vi "电信1801-2018012704-杜兴安-虚拟仪器作业5.vi"() -> ()   [LabVIEW 2020]
uses:
  <vilib>/Analysis/2dsp.llb/Real FFT.vi
  <vilib>/measure/matone.llb/Harmonic Distortion Analyzer 1 Chan.vi
  <vilib>/measure/mascope.llb/Cycle Average and RMS 1 chan.vi
  <vilib>/measure/NI_MABase.lvlib
  <vilib>/measure/NI_MAPro.lvlib
  <vilib>/Analysis/NI_AALPro.lvlib
  <vilib>/Analysis/NI_AALBase.lvlib
panel:
  out "谐波幅值":dbl[](array[numeric])
  out "检测的基频值":dbl
  out "THD%":dbl
  in  "谐波次数":dbl=4.0
  in  "采样点数 6":dbl=1000.0
  in  "采样频率 6":dbl=1000.0
  in  "基频":dbl=50.0
  out "频谱":T1(graph)
  out "信号波形 2":waveform(dbl)(graph)
  in  "采样点数 5":dbl=100.0
  in  "采样频率 5":dbl=100.0
  in  "信号频率 3":dbl=5.0
  out "相位谱波形":T2(graph)
  out "幅度谱波形":T3(graph)
  out "信号波形":waveform(dbl)(graph)
  out "实际单频信号频率":dbl[](array[numeric])
  in  "采样信息":cluster{"采样频率":dbl, "采样点数":dbl}={"采样频率"=1000.0, "采样点数"=1000.0}
  in  "初始相位 2":dbl[](array[numeric])
  in  "幅值 2":dbl[](array[numeric]) format="%02_2g"
  in  "频率 2":dbl[](array[numeric])
  out "波形图 4":waveform(dbl)(graph)
  in  "采样点数 4":dbl=100.0
  in  "采样频率 4":dbl=100.0
  in  "幅值2":dbl=2.0
  in  "频率2":dbl=20.0
  in  "幅值1":dbl=1.0
  in  "频率1":dbl=10.0
  out "频域波形":cluster{i32, dbl, dbl[]}(graph)
  out "时域波形":cluster{i32, dbl, dbl[]}(graph)
  out "波形图 3":waveform(dbl)(graph)
  in  "采样点数 3":dbl=1000.0
  in  "采样频率 3":dbl=1000.0
  in  "公式":string="sin(w*t)/(w*t)"
  in  "幅值":dbl=1.0
  in  "频率":dbl=5.0
  out "波形图 2":waveform(dbl)(graph)
  in  "信号频率 2":dbl=5.0
  in  "信号幅度":dbl=1.0
  in  "初始相位":dbl
  in  "方波占空比":dbl=50.0
  in  "采样频率 2":dbl=1000.0
  in  "采样点数 2":dbl=1000.0
  in  "信号类型":u16(ring) items=["正弦波", "三角波", "方波", "锯齿波"]
  in  "停止 2":bool
  in  "信号幅值":dbl=1.0
  in  "信号频率":dbl=5.0
  in  "采样频率":dbl=1000.0
  in  "采样点数":dbl=1000.0
  out "波形图":waveform(dbl)(graph)
  in  "停止":bool
  out "周期平均值":sgl format="%04_1f"
  out "周期均方根":sgl format="%04_3g"
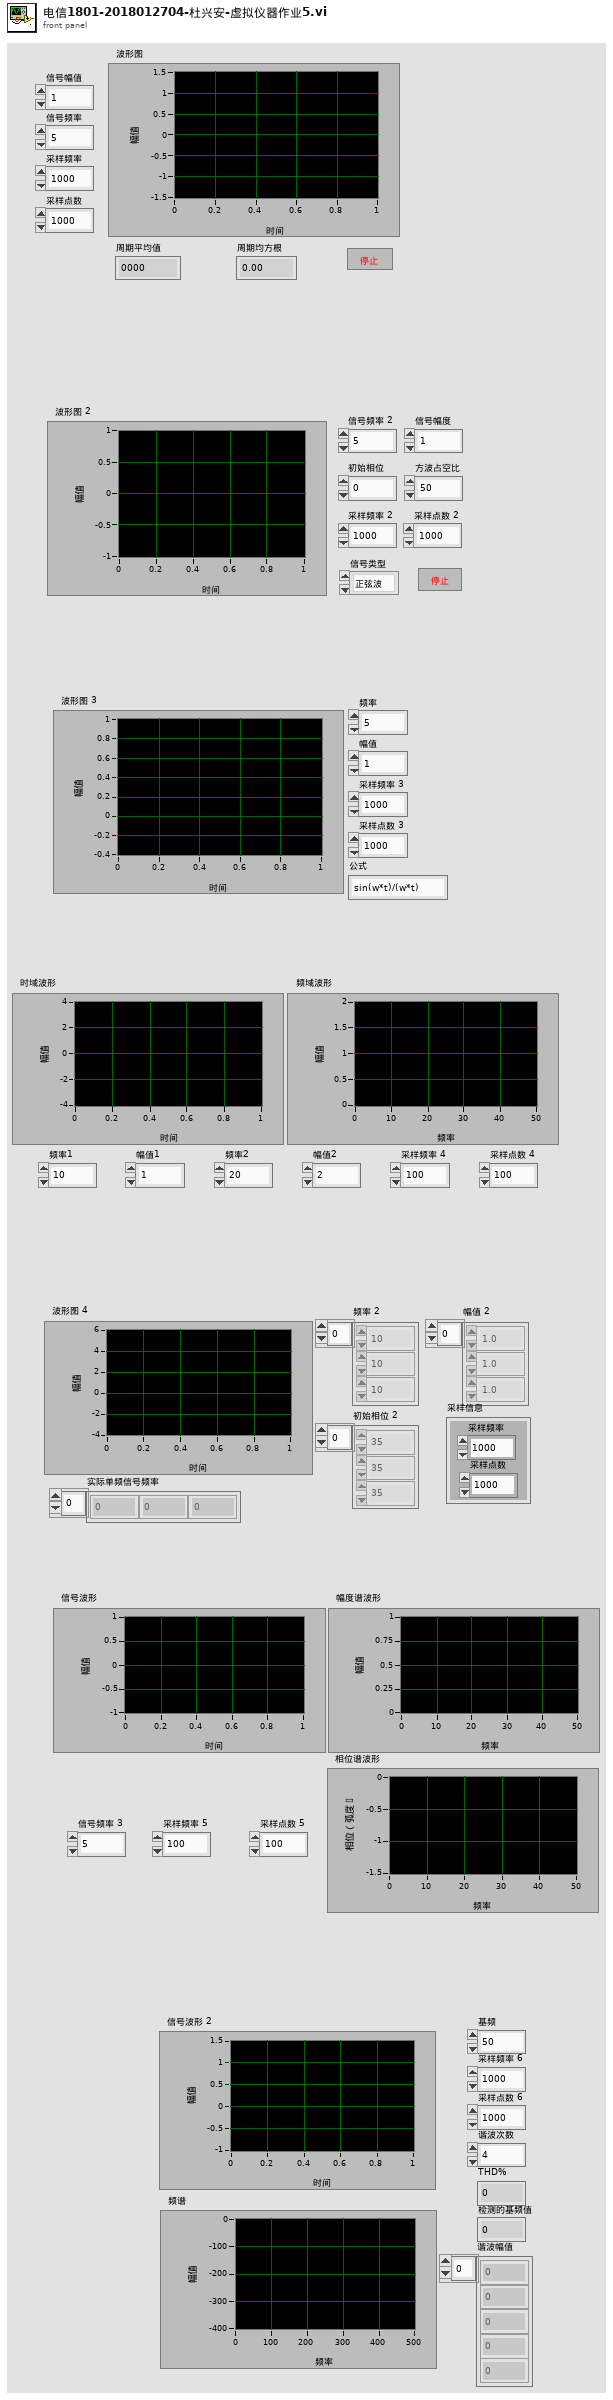
[diagram p1: front panel]
types:
  T1 = cluster{"f0":dbl, "df":dbl, "dB Spectrum (Hann)":dbl[]}
  T2 = cluster{i32, "df":dbl, "Amp Spectrum Phase (radians)":dbl[]}
  T3 = cluster{i32, "df":dbl, "Amp Spectrum Mag (Vrms)":dbl[]}
  T4 = enum16{"none", "input signal", "fundamental signal", "residual signal", "harmonics only", "noise and spurs"}
  T5 = cluster{"exported time signal":waveform(dbl), "exported spectrum (dB)":cluster{"f0":dbl, "df":dbl, "dB Spectrum (Hann)":dbl[]}}
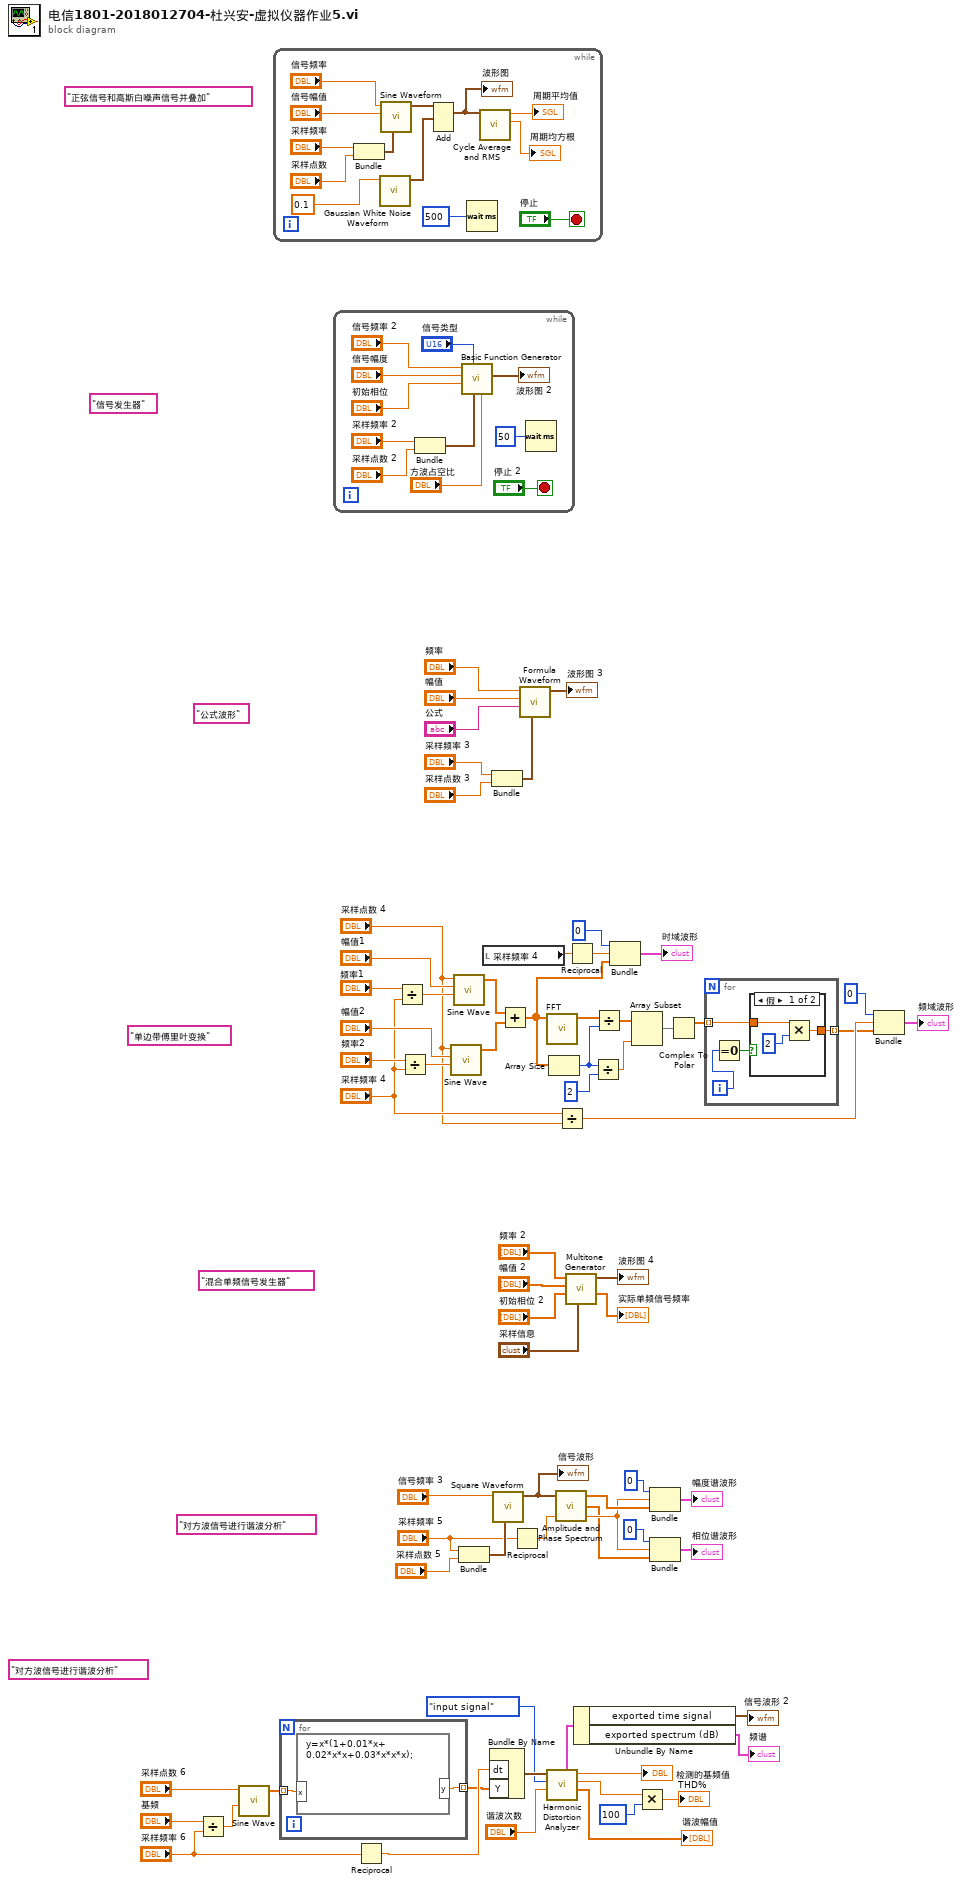
[diagram p0: block diagram]
diagram:
  (unwired) "对方波信号进行谐波分析"
  (unwired) "混合单频信号发生器"
  (unwired) "对方波信号进行谐波分析"
  (unwired) "单边带傅里叶变换"
  (unwired) "公式波形"
  (unwired) "信号发生器"
  (unwired) "正弦信号和高斯白噪声信号并叠加"
  n1 = Divide(x="基频", y="采样频率 6") -> (x/y=w16:dbl)
  n2 = call <vilib>:"Sine Wave.vi"("samples"="采样点数 6", "frequency"=w16) -> ("sine wave"=w15:dbl[])  [unwired: 3 in, 2 out]
  n3 = while {
    stop <- "停止" stop-if-true
    n4 = Bundle("采样频率"="采样频率", "采样点数"="采样点数") -> (w78:cluster{"采样频率":dbl, "采样点数":dbl})  [unwired: 1 in]
    n5 = call <vilib>:"Gaussian White Noise Waveform.vi"("standard deviation"=0.1) -> ("signal out"=w75:waveform(dbl))  [unwired: 9 in, 1 out]
    n6 = call <vilib>:"Sine Waveform.vi"("sampling info"=w78, "amplitude"="信号幅值", "frequency"="信号频率") -> ("signal out"=w76:waveform(dbl))  [unwired: 7 in, 1 out]
    n7 = Add(1:w75, 2:w76) -> (0:w74:waveform(dbl))  [unwired: 1 in, 1 out]
    "波形图" <- w74
    n8 = Wait (ms)(milliseconds to wait=500) -> ()  [unwired: 1 out]
    n9 = call-poly <vilib>:"Cycle Average and RMS.vi"("signal in"=w74) -> ("cycle RMS"=→"周期均方根":dbl, "cycle average"=→"周期平均值":dbl)  [unwired: 7 in, 2 out]
  }
  n10 = for {
    tunnel: w15 -> [w85] mode=indexing
    tunnel: [w84] -> w12 mode=indexing
    n11 = formula code="y=x*(1+0.01*x+\n0.02*x*x+0.03*x*x*x);"("x"=w85) -> ("y"=w84:dbl)
  }
  n12 = while {
    stop <- "停止 2" stop-if-true
    n13 = Bundle("采样频率 2"="采样频率 2", "采样点数 2"="采样点数 2") -> (w94:cluster{"采样频率 2":dbl, "采样点数 2":dbl})  [unwired: 1 in]
    n14 = call <vilib>:"Basic Function Generator.vi"("square wave duty cycle (%)"="方波占空比", "sampling info"=w94, "signal type"="信号类型", "phase"="初始相位", "amplitude"="信号幅度", "frequency"="信号频率 2") -> ("signal out"=→"波形图 2":waveform(dbl))  [unwired: 3 in, 2 out]
    n15 = Wait (ms)(milliseconds to wait=50) -> ()  [unwired: 1 out]
  }
  n16 = Reciprocal(x="采样频率 6") -> (1/x=w13:dbl)
  n17 = Divide(x="频率1", y="采样频率 4") -> (x/y=w60:dbl)
  n18 = Divide(x="频率2", y="采样频率 4") -> (x/y=w61:dbl)
  n19 = call <vilib>:"Sine Wave.vi"("samples"="采样点数 4", "amplitude"="幅值2", "frequency"=w61) -> ("sine wave"=w56:dbl[])  [unwired: 2 in, 2 out]
  n20 = call <vilib>:"Sine Wave.vi"("samples"="采样点数 4", "amplitude"="幅值1", "frequency"=w60) -> ("sine wave"=w57:dbl[])  [unwired: 2 in, 2 out]
  n21 = Bundle("采样频率 5"="采样频率 5", "采样点数 5"="采样点数 5") -> (w29:cluster{"采样频率 5":dbl, "采样点数 5":dbl})  [unwired: 1 in]
  n22 = local read "采样频率 4"() -> (w54:dbl)
  n23 = Bundle By Name("dt"=w13, "Y"=w12) -> (w11:waveform(dbl))  [unwired: 1 in]
  n24 = Bundle("采样频率 3"="采样频率 3", "采样点数 3"="采样点数 3") -> (w65:cluster{"采样频率 3":dbl, "采样点数 3":dbl})  [unwired: 1 in]
  n25 = call <vilib>:"Square Waveform.vi"("sampling info"=w29, "frequency"="信号频率 3") -> ("signal out"=w19:waveform(dbl))  [unwired: 8 in, 1 out]
  "信号波形" <- w19
  n26 = Add(x=w57, y=w56) -> (x+y=w51:dbl[])
  n27 = Reciprocal(x="采样频率 5") -> (1/x=w28:dbl)
  n28 = call <vilib>:"Formula Waveform.vi"("sampling info"=w65, "formula"="公式", "amplitude"="幅值", "frequency"="频率") -> ("signal out"=→"波形图 3":waveform(dbl))  [unwired: 6 in, 1 out]
  n29 = call-poly <vilib>:"FFT.vi"("X"=w51) -> ("FFT {X}"=w50:cdb[])  [unwired: 9 in, 1 out]
  n30 = call-poly <vilib>:"Harmonic Distortion Analyzer.vi"("highest harmonic"="谐波次数", "export mode"=T4."input signal", "signal in"=w11) -> ("components level"=→"谐波幅值":dbl[], "THD"=w3:dbl, "detected fundamental frequency"=→"检测的基频值":dbl, "exported signals"=w8:T5)  [unwired: 3 in, 2 out]
  n31 = Array Size(array=w51) -> (size(s)=w44:i32)
  n32 = call <vilib>:"Amplitude and Phase Spectrum.vi"("dt"=w28, "Signal (V)"=w19) -> ("df"=w23:dbl, "Amp Spectrum Phase (radians)"=w22:dbl[], "Amp Spectrum Mag (Vrms)"=w25:dbl[])  [unwired: 1 in]
  n33 = Divide(x="采样频率 4", y="采样点数 4") -> (x/y=w48:dbl)
  n34 = call <vilib>:"Multitone Generator.vi"("sampling info"="采样信息", "tone phases"="初始相位 2", "tone amplitudes"="幅值 2", "tone frequencies"="频率 2") -> ("actual tone frequencies"=→"实际单频信号频率":dbl[], "signal out"=→"波形图 4":waveform(dbl))  [unwired: 4 in, 2 out]
  n35 = Reciprocal(x=w54) -> (1/x=w53:dbl)
  n36 = Unbundle By Name(w8) -> ("exported time signal"=→"信号波形 2":waveform(dbl), "exported spectrum (dB)"=→"频谱":T1)
  n37 = Divide(x=w44, y=2) -> (x/y=w41:dbl)
  n38 = Divide(x=w50, y=w44) -> (x/y=w42:cdb[])
  n39 = Bundle(0, w53, w51) -> (→"时域波形":cluster{i32, dbl, dbl[]})  [unwired: 1 in]
  n40 = Array Subset(array=w42, length=w41) -> (w40:cdb[])  [unwired: 1 in]
  n41 = Multiply(x=w3, y=100) -> (x*y=→"THD%":dbl)
  n42 = Bundle(0, "df"=w23, "Amp Spectrum Mag (Vrms)"=w25) -> (→"幅度谱波形":T3)  [unwired: 1 in]
  n43 = Bundle(0, "df"=w23, "Amp Spectrum Phase (radians)"=w22) -> (→"相位谱波形":T2)  [unwired: 1 in]
  n44 = Complex To Polar(r * e^(i*theta)=w40) -> (r=w39:dbl[])  [unwired: 1 out]
  n45 = for {
    tunnel: w39 -> [w98] mode=indexing
    tunnel: [w97] -> w38 mode=indexing
    i -> [w99]
    n46 = Equal To 0?(x=w99) -> (x = 0?=w100:bool)
    n47 = case shown="假" w100 {
      tunnel: w98 -> [w102 w104]
      tunnel: [w101 w104] -> w97
      frame False {
        n48 = Multiply(x=w102, y=2) -> (x*y=w101:dbl)
      }
      frame True {
      }
    }
  }
  n49 = Bundle(0, w48, w38) -> (→"频域波形":cluster{i32, dbl, dbl[]})  [unwired: 1 in]
